vi "LBNE_Global .vi"() -> ()   [LabVIEW 2014]
uses:
  D:/share/LIQ_ARG/LBNE_SW/LBNE_DLL/LBNE_DLL/bin/Debug/LBNE_DLL.dll
  LBNE_DLL/LBNE_DLL/bin/Debug/LBNE_DLL.dll
panel:
  out "UDP/I2C":bool=TRUE
  out "LBNE_REF":refnum<k24>
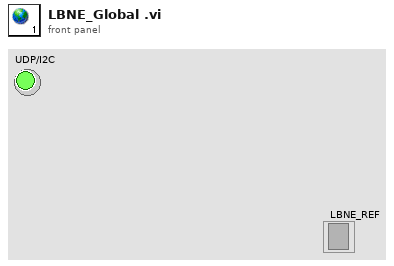
[diagram p1: front panel]
diagram:
